vi "Browse for XNET Database.vi"(8 "error in (no error)":errorcluster) -> (0 "error out":errorcluster, 2 "Cancel Out":bool, 3 "XNET Settings":T1={"Database"="", "Cluster"="", "Primary"={"Port"="", "Baud Rate"=0, "Termination"=0, "CAN I/O Mode"=0, "FD Baud Rate"=500000, "Priority"=100, "FD ISO Mode"=0}, "Ghost"={"Port"="", "Baud Rate"=0, "Termination"=0, "CAN I/O Mode"=0, "FD Baud Rate"=500000, "Priority"=100, "FD ISO Mode"=0}} {"Ghost"."FD ISO Mode" items=["ISO", "Non ISO", "ISO Legacy"]; "Ghost"."CAN I/O Mode" items=["CAN 2.0", "CAN FD", "CAN FD+BRS"]; "Ghost"."Termination" items=["Off", "On"]; "Primary"."FD ISO Mode" items=["ISO", "Non ISO", "ISO Legacy"]; "Primary"."CAN I/O Mode" items=["CAN 2.0", "CAN FD", "CAN FD+BRS"]; "Primary"."Termination" items=["Off", "On"]})   [LabVIEW 2019, in "Ghost Bus Addon System Explorer.lvlib"]
uses:
  Ghost Bus Addon System Explorer.lvlib
  <resource>/objmgr/xnet.rc
  Addon Shared/Types/XNET Settings.ctl
  Addon Shared/Ghost Bus Addon Shared.lvlib
  Addon Shared/Types/XNET Port Settings.ctl
panel:
  in  "FD Baud rate [Bd]":u64=500000
  out "CAN I/O Mode":u32(ring) items=["CAN 2.0", "CAN FD", "CAN FD+BRS"]
  in  "Baud rate [Bd]":u64=500000
  in  "Select CAN Cluster":u16(ring)
  in  "Cancel":bool
  in  "Select":bool
  in  "XNET Database":refnum<k21>
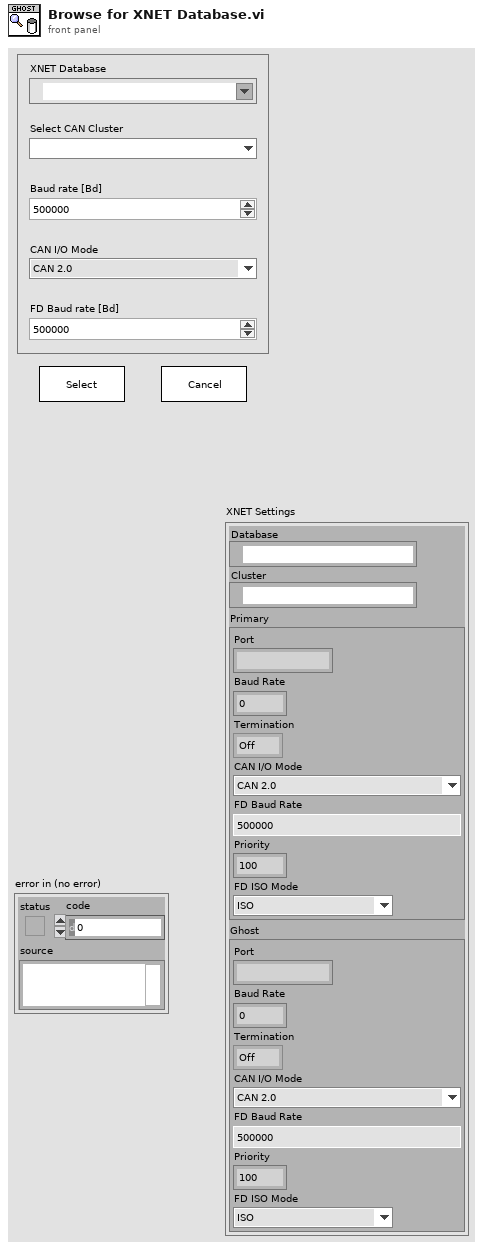
[diagram p1: front panel]
types:
  T1 = typedef "Ghost Bus Addon Shared.lvlib/XNET Settings.ctl" = cluster{"Database":refnum<k21>, "Cluster":refnum<k21>, "Primary":T2, "Ghost":T2}
  T2 = typedef "Ghost Bus Addon Shared.lvlib/XNET Port Settings.ctl" = cluster{"Port":string, "Baud Rate":u64, "Termination":u32, "CAN I/O Mode":u32, "FD Baud Rate":u64, "Priority":i32, "FD ISO Mode":u32}
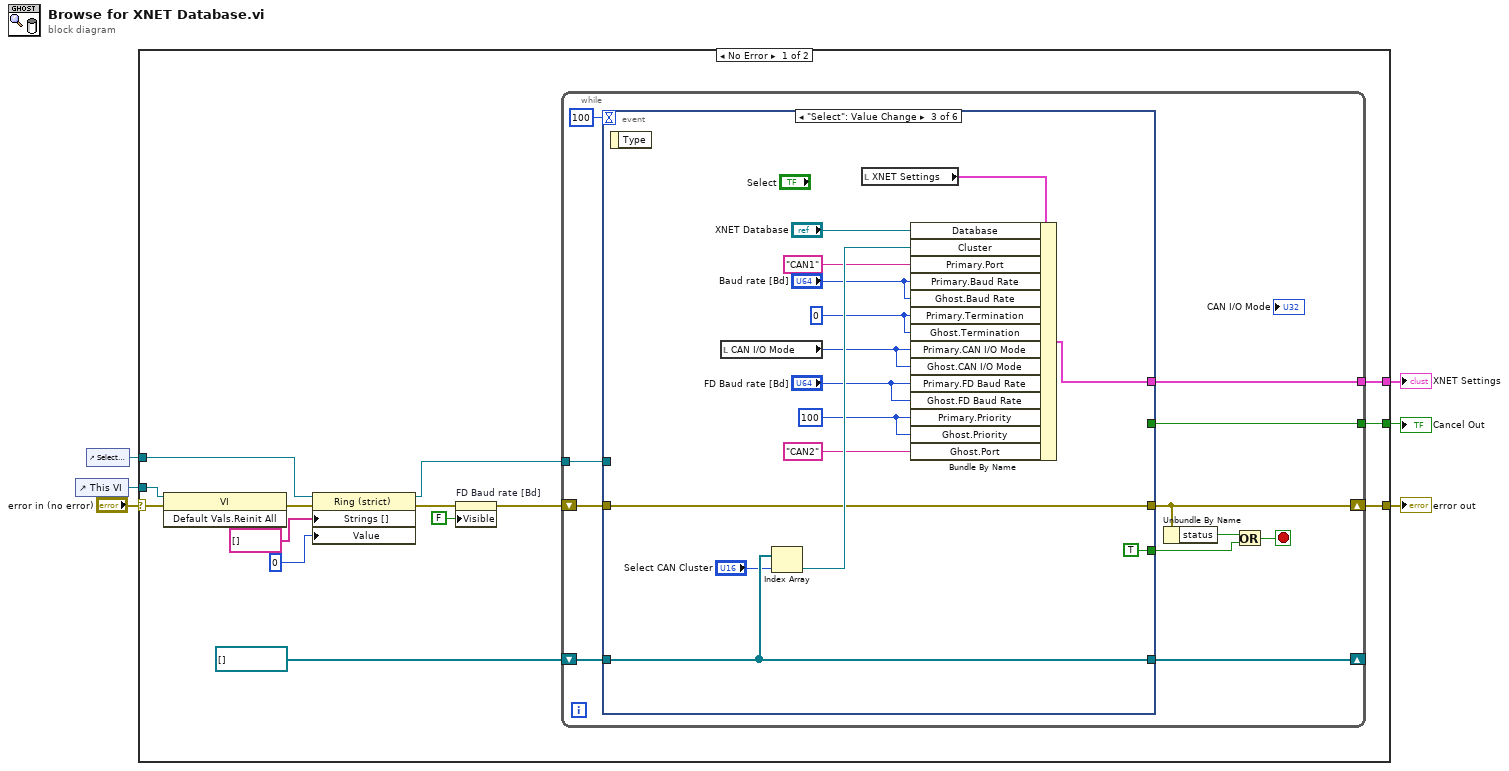
[diagram p0: block diagram]
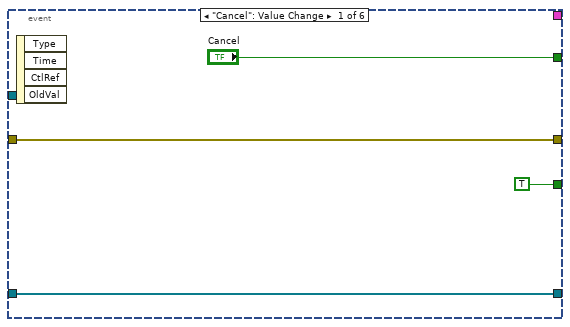
[diagram p2: hidden frame]
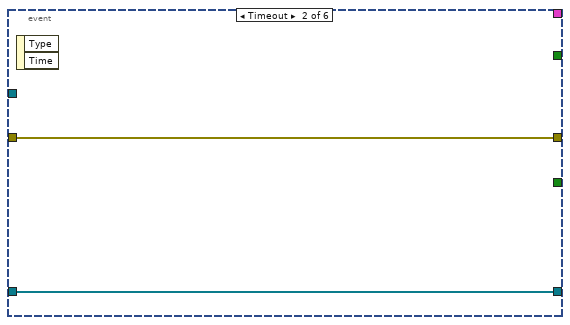
[diagram p3: hidden frame]
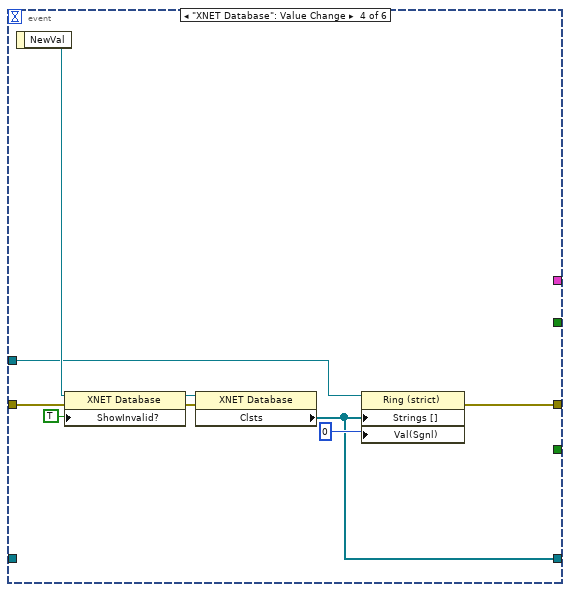
[diagram p4: hidden frame]
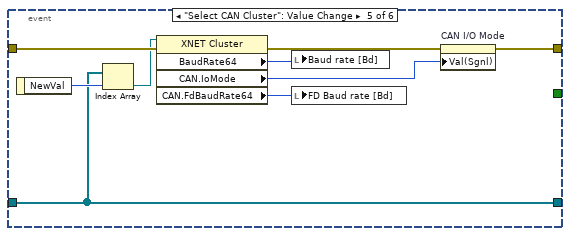
[diagram p5: hidden frame]
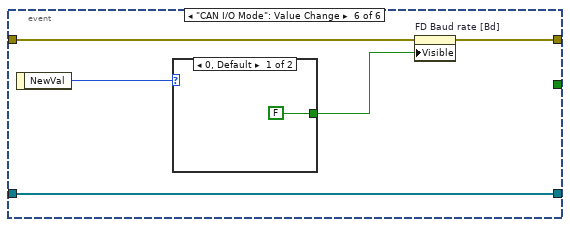
[diagram p6: hidden frame]
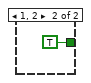
[diagram p7: hidden frame]
diagram:
  n1 = control-ref of="This VI"() -> (w3:refnum<vi>)
  n2 = control-ref of="Select CAN Cluster"() -> (w1:refnum<vi>)
  n3 = case shown="No Error" "error in (no error)" {
    selector: "error in (no error)" -> [w19 w78]
    tunnel: [w17 w78] -> w5
    tunnel: [w20 _] -> w4
    tunnel: w3 -> [w18 _]
    tunnel: [w15 _] -> w2
    tunnel: w1 -> [w14 _]
    frame No Error {
      n4 = invoke class="VI" method="Default Vals.Reinit All"(reference=w18, error in=w19) -> (error out=w13:errorcluster)  [unwired: 1 in, 2 out]
      n5 = property on="Property Node" class="Ring (strict)"(reference=w14, error in=w13, "Strings []"=string[] [], "Value"=u16 0) -> (reference out=w12:refnum<vi>, error out=w9:errorcluster)
      n6 = property on="FD Baud rate [Bd]" class="DigNum (strict)"(error in=w9, "Visible"=FALSE) -> (error out=w8:errorcluster)  [unwired: 1 in, 1 out]
      n7 = while {
        tunnel: [w31] -> w20
        shift-right: [w29] -> _
        shift-left: refnum<k21>[] [] ("Clsts") -> [w28]
        shift-right: [w25] -> w17
        shift-left: w8 -> [w30]
        tunnel: [w27] -> w15
        tunnel: w12 -> [w21]
        stop <- w22 stop-if-true
        n8 = event shown="[2] \"Select\": Value Change" {
          selector: _ -> [_ _ _ _ _ _]
          dyn-events: _ -> [_ _ _ _ _ _]
          timeout: 100 -> [_ _ _ _ _ _]
          tunnel: ["Cancel" _ _ _ _ _] -> w31
          tunnel: w30 -> [w33 w37 w46 w58 w69 w75]
          tunnel: [w34 w36 w50 w55 w66 w73] -> w29
          tunnel: w28 -> [w34 w36 w50 _ w66 w73]
          tunnel: [w33 w37 w46 w53 w64 w74] -> w25
          tunnel: [_ _ w47 _ _ _] -> w27
          tunnel: [TRUE _ TRUE _ _ _] -> w23
          tunnel: w21 -> [_ _ _ w54 _ _]
          event "Cancel": Value Change {
            n9 = event-data() -> ()  [unwired: 1 in, 4 out]
          }
          event Timeout {
            n10 = event-data() -> ()  [unwired: 1 in, 2 out]
          }
          event "Select": Value Change {
            w42 = 100 ("Priority")
            w43 = u32 0 ("Termination")
            n11 = event-data() -> ()  [unwired: 1 in, 1 out]
            n12 = local read "CAN I/O Mode"() -> (w40:u32)
            n13 = Index Array(array=w50, index="Select CAN Cluster") -> (element=w48:refnum<k21>)
            n14 = local read "XNET Settings"() -> (w51:T1)
            n15 = Bundle By Name(cluster=w51, "Database"="XNET Database", "Cluster"=w48, "Primary.Port"="CAN1" ("Port"), "Primary.Baud Rate"="Baud rate [Bd]", "Ghost.Baud Rate"="Baud rate [Bd]", "Primary.Termination"=w43, "Ghost.Termination"=w43, "Primary.CAN I/O Mode"=w40, "Ghost.CAN I/O Mode"=w40, "Primary.FD Baud Rate"="FD Baud rate [Bd]", "Ghost.FD Baud Rate"="FD Baud rate [Bd]", "Primary.Priority"=w42, "Ghost.Priority"=w42, "Ghost.Port"="CAN2" ("Port")) -> (w47:T1)
          }
          event "XNET Database": Value Change {
            n16 = event-data() -> ("NewVal"=w57:refnum<k21>)  [unwired: 1 in]
            n17 = property class="XNET Database"(reference=w57, error in=w58, "ShowInvalid?"=TRUE ("Show Invalid From Open?")) -> (reference out=w61:refnum<k21>, error out=w60:errorcluster)
            n18 = property class="XNET Database"(reference=w61, error in=w60) -> ("Clsts"=w55:refnum<k21>[])  [unwired: 2 out]
            n19 = property on="Property Node" class="Ring (strict)"(reference=w54, "Strings []"=w55, "Val(Sgnl)"=u16 0 ("Value (Signaling)")) -> (error out=w53:errorcluster)  [unwired: 1 in, 1 out]
          }
          event "Select CAN Cluster": Value Change {
            n20 = event-data() -> ("NewVal"=w68:u16)  [unwired: 1 in]
            n21 = Index Array(array=w66, index=w68) -> (element=w67:refnum<k21>)
            n22 = property class="XNET Cluster"(reference=w67, error in=w69) -> (error out=w63:errorcluster, "BaudRate64"=w70:u64, "CAN.IoMode"=w62:u32, "CAN.FdBaudRate64"=w65:u64)  [unwired: 1 out]
            n23 = local write "Baud rate [Bd]"(w70) -> ()
            n24 = local write "FD Baud rate [Bd]"(w65) -> ()
            n25 = property on="CAN I/O Mode" class="Ring (strict)"(error in=w63, "Val(Sgnl)"=w62) -> (error out=w64:errorcluster)  [unwired: 1 in, 1 out]
          }
          event "CAN I/O Mode": Value Change {
            n26 = event-data() -> ("NewVal"=w71:u32)  [unwired: 1 in]
            n27 = case shown="0, Default" w71 {
              tunnel: [FALSE TRUE] -> w72
              frame 0, Default {
              }
              frame 1, 2 {
              }
            }
            n28 = property on="FD Baud rate [Bd]" class="DigNum (strict)"(error in=w75, "Visible"=w72) -> (error out=w74:errorcluster)  [unwired: 1 in, 1 out]
          }
        }
        n29 = Unbundle By Name(w25) -> ("status"=w24:bool)
        n30 = Or(x=w24, y=w23) -> (x .or. y?=w22:bool)
      }
    }
    frame Error {
    }
  }
  "error out" <- w5
  "Cancel Out" <- w4
  "XNET Settings" <- w2
